vi "ServiceSendProperties.vi"   [LabVIEW 2015]
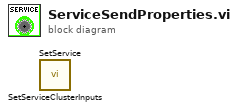
[diagram p0: block diagram]
diagram:
  n1 = call "SetServiceClusterInputs.vi"() -> ()  [unwired: 10 in, 2 out]
  n2 = call "SetService.vi"() -> ()  [unwired: 10 in, 2 out]
